vi "Raise Error.vi"(8 "Error In":errorcluster, 11 "Error":T1) -> (0 "Error Out":errorcluster)   [LabVIEW 2011, in "Tinkerforge.lvlib" / "IP Connection.lvclass"]
doc: "This VI raises an error with a complete call chain."
uses:
  IP Connection.lvclass
  Type Definitions/Errors.ctl
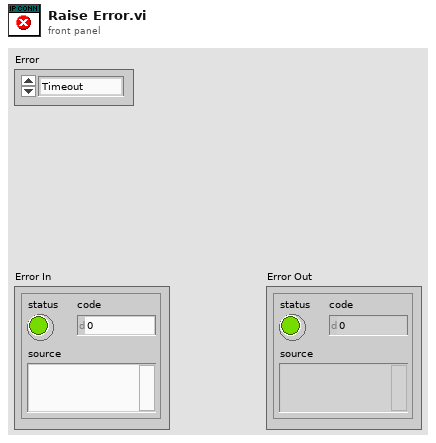
[diagram p1: front panel]
types:
  T1 = typedef "Tinkerforge.lvlib/IP Connection.lvclass/Errors.ctl" = enum16{"Timeout", "Device type incorrect", "Device already added", "Device not existing"}
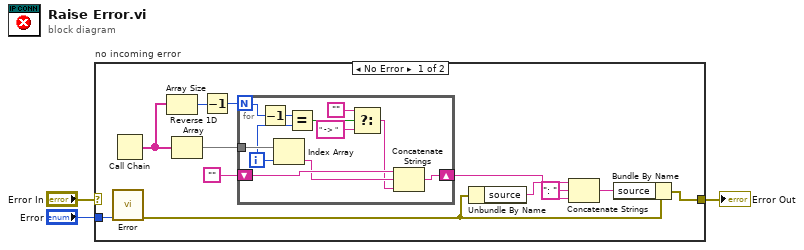
[diagram p0: block diagram]
diagram:
  n1 = case "no incoming error" shown="No Error" "Error In" {
    selector: "Error In" -> [_ w27]
    tunnel: [w9 w27] -> w2
    tunnel: "Error" -> [w15 _]
    frame No Error {
      n2 = call "Error.vi"("Error"=w15) -> ("error cluster"=w8:errorcluster)  [unwired: 10 in]
      n3 = Call Chain() -> (call chain=w13:string[])
      n4 = Array Size(array=w13) -> (size(s)=w12:i32)
      n5 = Reverse 1D Array(array=w13) -> (reversed array=w10:string[])
      n6 = Decrement(x=w12) -> (x-1=w14:i32)
      n7 = for {
        N: w14 -> [w22]
        tunnel: w10 -> [w26]
        shift-right: [w25] -> w5
        shift-left: "" -> [w24]
        i -> [w20]
        n8 = Decrement(x=w22) -> (x-1=w21:i32)
        n9 = Index Array(array=w26, index=w20) -> (element=w23:string)
        n10 = Equal?(x=w21, y=w20) -> (x = y?=w19:bool)
        n11 = Select(t="", s=w19, f=" -> " ("string")) -> (s? t:f=w16:string)
        n12 = Concatenate Strings(w24, w23, w16) -> (w25:string)
      }
      n13 = Unbundle By Name(w8) -> ("source"=w7:string)
      n14 = Concatenate Strings(w7, ": " ("string"), w5) -> (w4:string)
      n15 = Bundle By Name(cluster=w8, "source"=w4) -> (w9:errorcluster)
    }
    frame Error {
    }
  }
  "Error Out" <- w2
